vi "logCtrlEllipse.vi"(0 "EllipsePath":path, 1 "time":dbl, 2 "eta_i":dbl[](array[numeric]), 3 "eta_r":dbl[](array[numeric]), 4 "e_i":cdb, 5 "e_psi":dbl) -> ()   [LabVIEW 2014]
uses:
  <vilib>/Utility/file.llb/Write To Spreadsheet File (DBL).vi
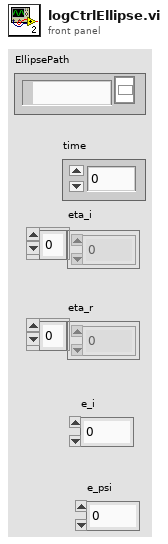
[diagram p1: front panel]
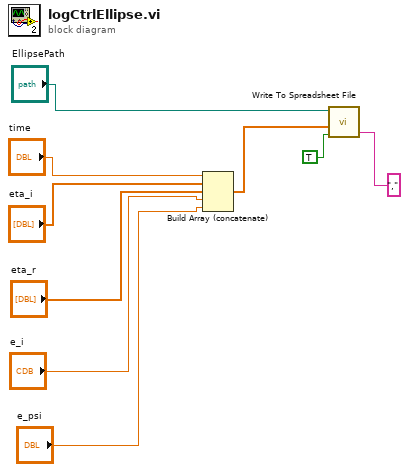
[diagram p0: block diagram]
diagram:
  n1 = Build Array (concatenate)("time", "eta_i", "eta_r", "e_i", "e_psi") -> (w9:cdb[])
  n2 = call-poly <vilib>:"Write To Spreadsheet File.vi"("delimiter (\\t)"="," ("delimiter (\\t)"), "append to file? (new file:F)"=TRUE, "1D data"=w9, "file path (dialog if empty)"="EllipsePath") -> ()  [unwired: 4 in, 1 out]
